vi "Tic Tac Toe - Without Event.vi"() -> ()   [LabVIEW 2022 SP3]
panel:
  in  "B 9":bool
  in  "B 8":bool
  in  "B 7":bool
  in  "B 6":bool
  in  "B 5":bool
  in  "B 4":bool
  in  "B 3":bool
  in  "B 2":bool
  in  "B 1":bool
  in  "Exit":bool
  in  "Reset":bool
  in  "Start Game":bool
  out "Player 2 Symbol":u16(ring)
  in  "Player 2 Name":string="Steve"
  out "Player 1 Symbol":u16(ring)
  in  "Player 1 Name":string="Mark"
  in  "9":u16(ring)
  in  "8":u16(ring)
  in  "7":u16(ring)
  in  "6":u16(ring)
  in  "5":u16(ring)
  in  "4":u16(ring)
  in  "3":u16(ring)
  in  "2":u16(ring)
  in  "1":u16(ring)
  # "TIC TAC TOE"
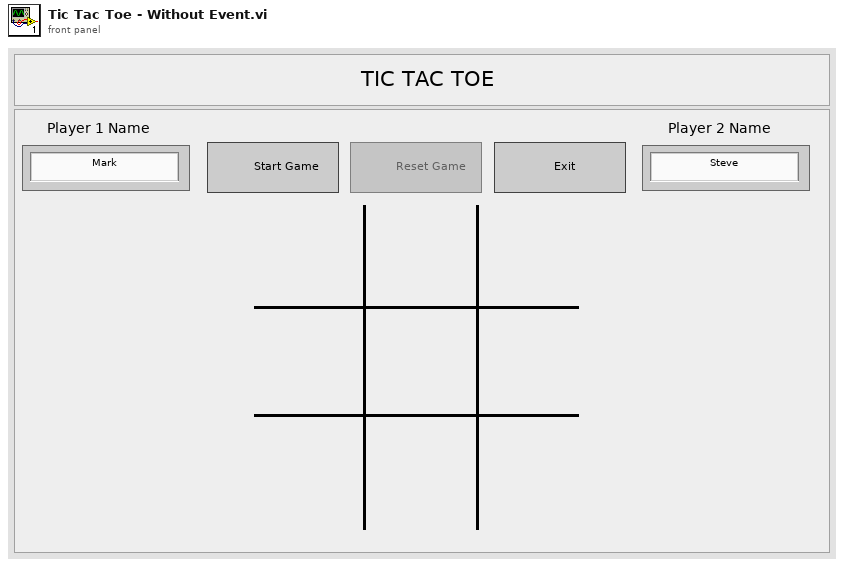
[diagram p1: front panel]
types:
  T1 = enum8{"Enabled", "Disabled", "Disabled and Grayed Out"}
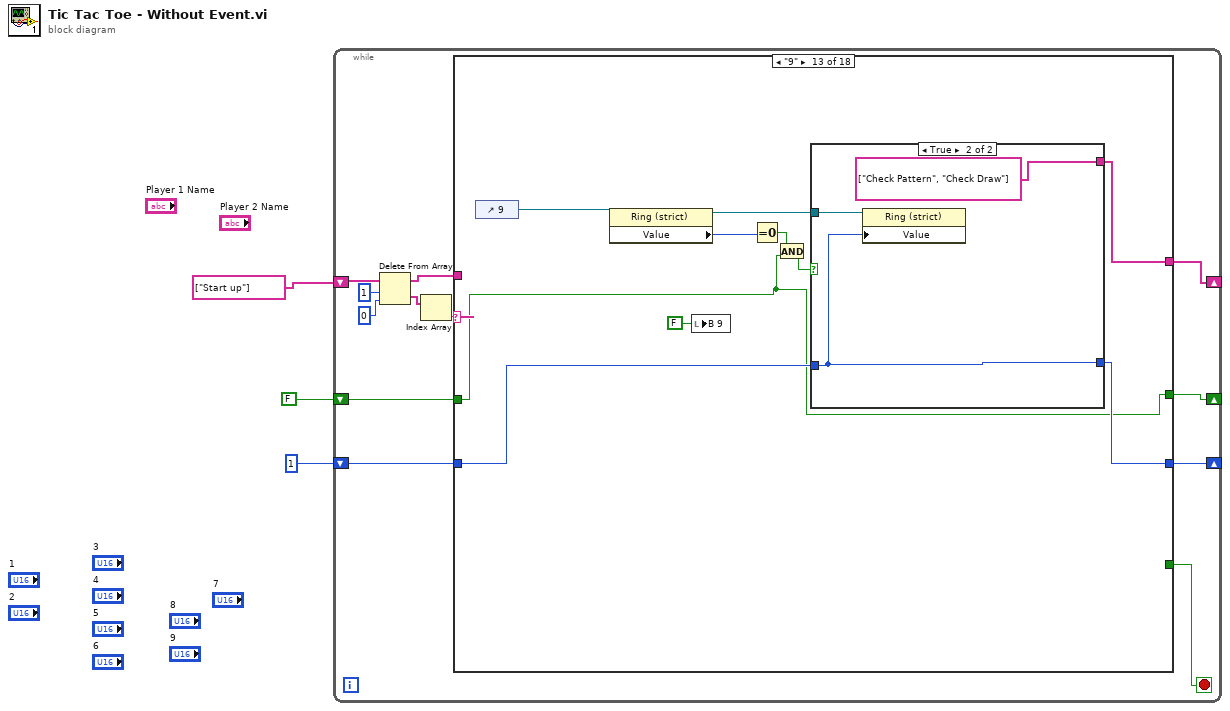
[diagram p0: block diagram]
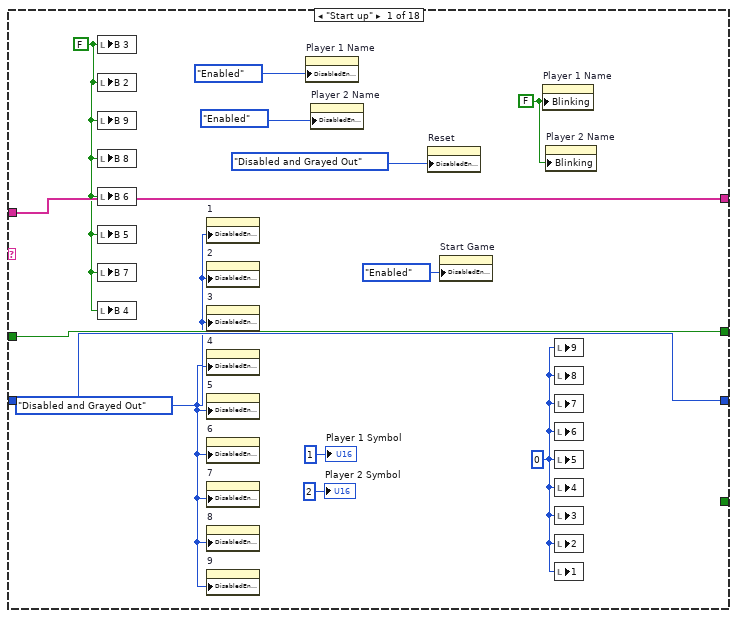
[diagram p2: hidden frame]
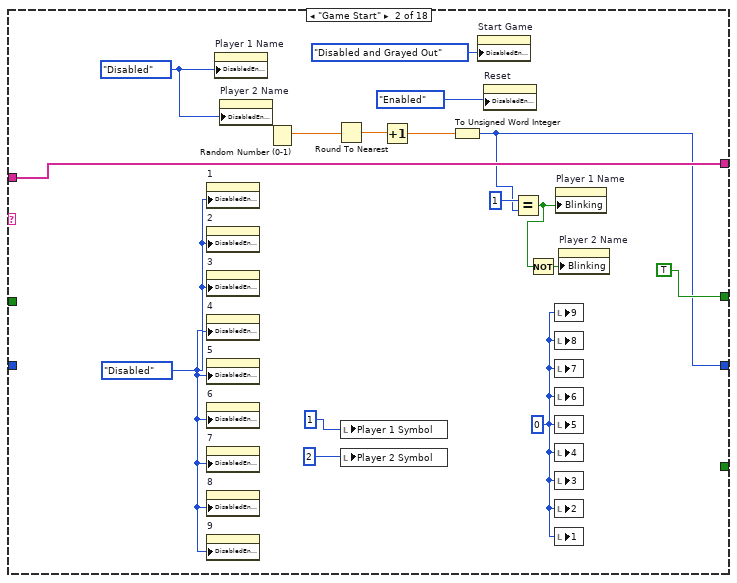
[diagram p3: hidden frame]
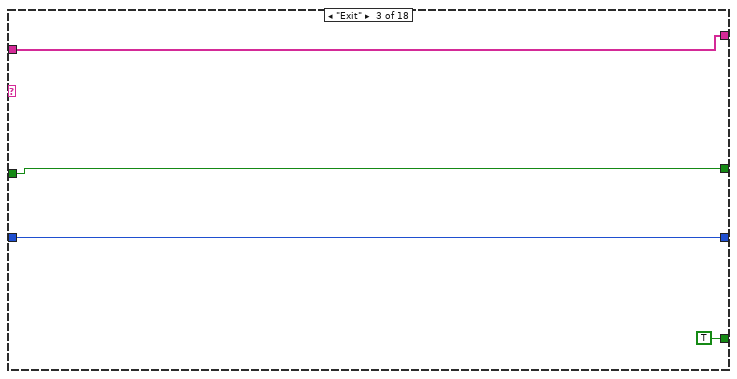
[diagram p4: hidden frame]
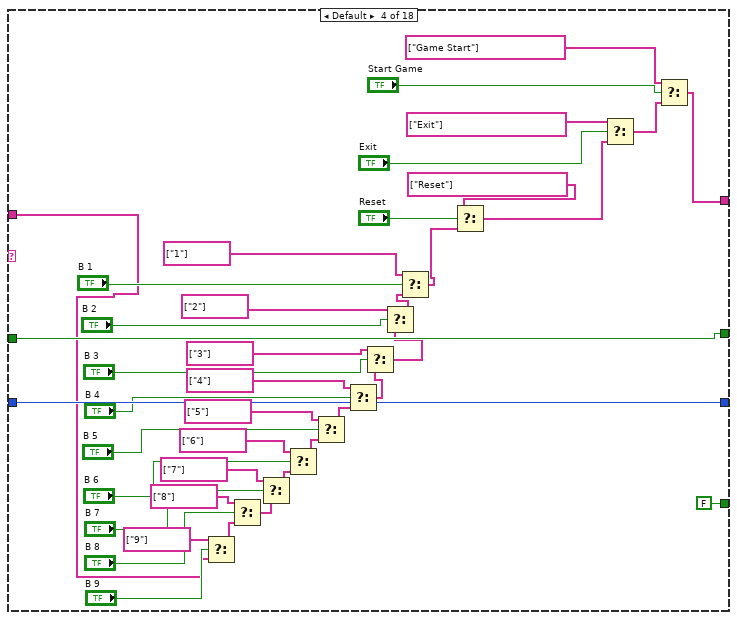
[diagram p5: hidden frame]
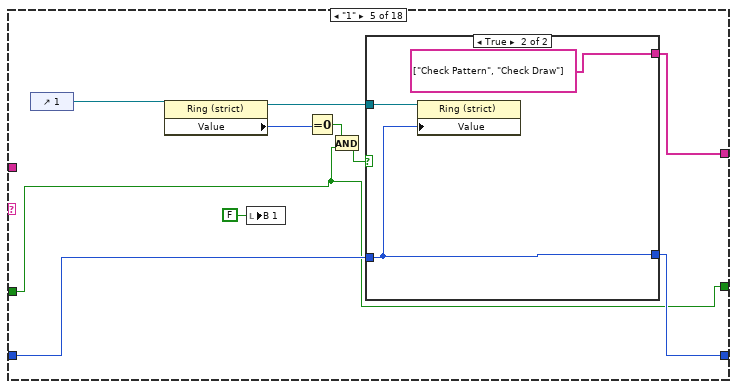
[diagram p6: hidden frame]
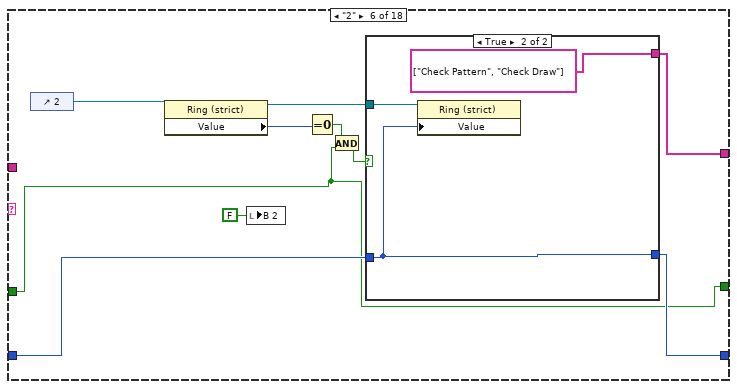
[diagram p8: hidden frame]
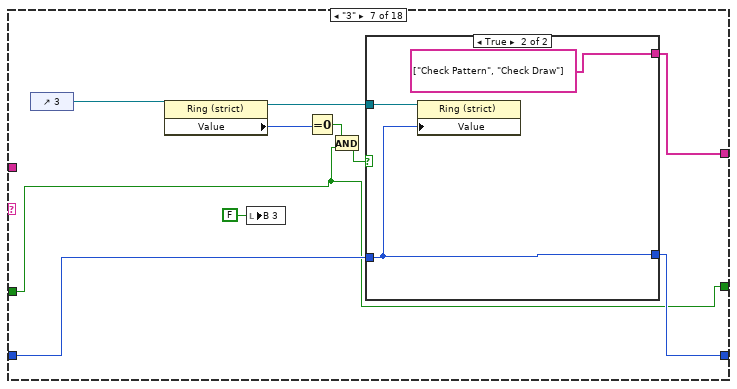
[diagram p10: hidden frame]
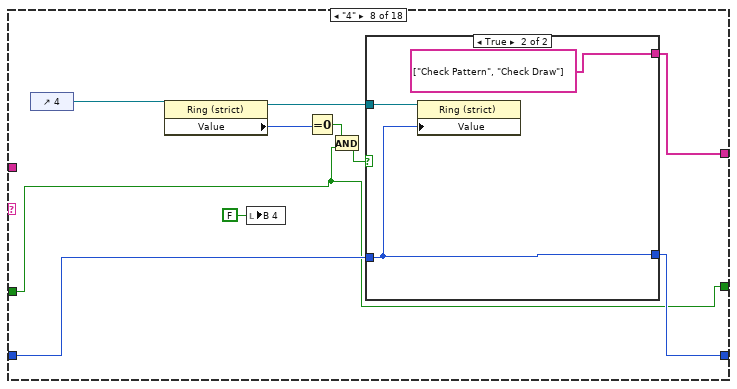
[diagram p12: hidden frame]
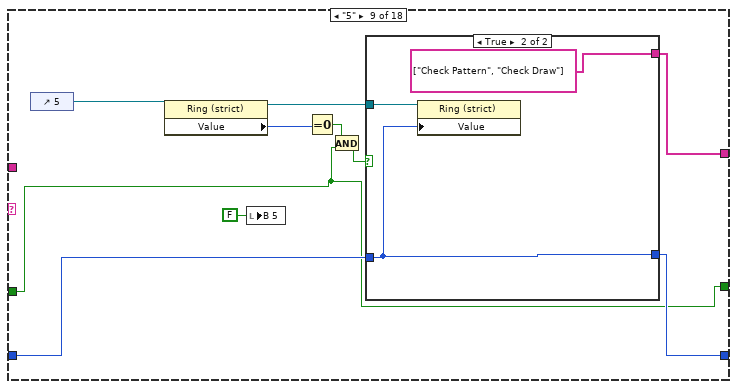
[diagram p14: hidden frame]
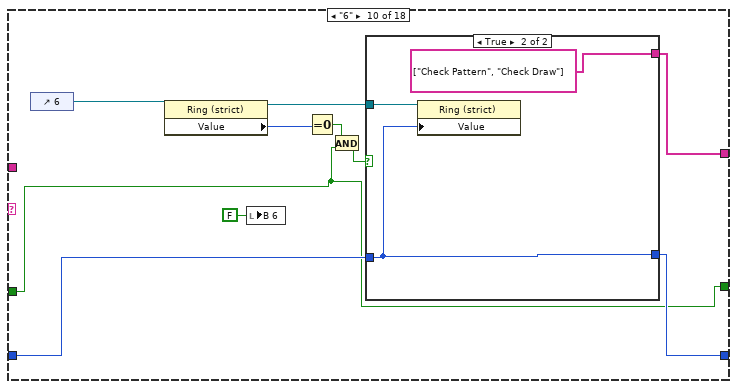
[diagram p16: hidden frame]
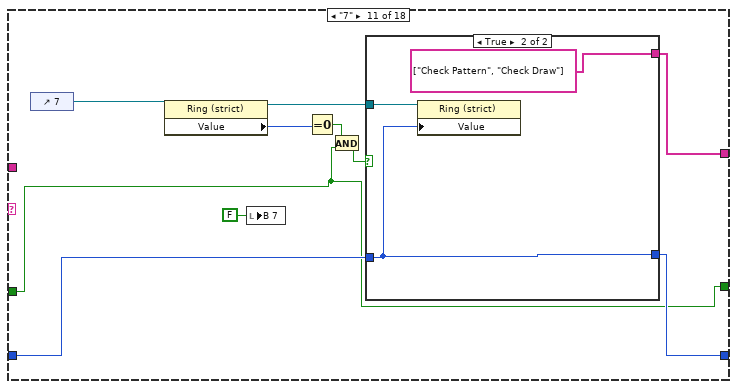
[diagram p18: hidden frame]
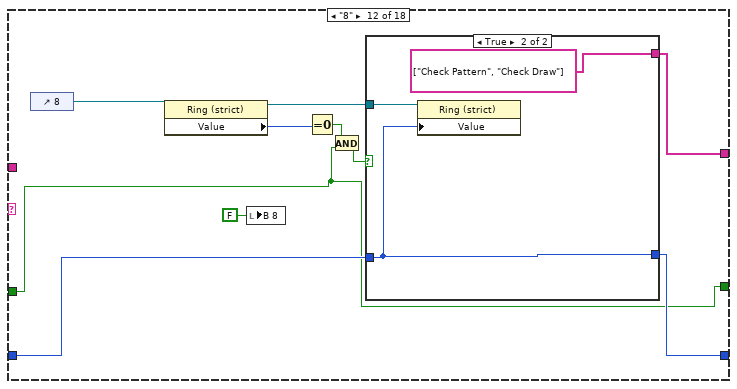
[diagram p20: hidden frame]
diagram:
  n1 = while {
    shift-right: [w10] -> _
    shift-left: string[] ["Start up"] -> [w15]
    shift-right: [w8] -> _
    shift-left: FALSE -> [w7]
    shift-right: [w6] -> _
    shift-left: u16 1 ("9") -> [w5]
    stop <- w4 stop-if-true
    n2 = Delete From Array(array=w15, length=1, index=0) -> (deleted portion=w12:string[], array with subset deleted=w9:string[])
    n3 = Index Array(array=w12) -> (element=w11:string)  [unwired: 1 in]
    n4 = case shown="\"9\"" w11 {
      tunnel: [w28 w44 w45 w83 w94 w108 w122 w136 w150 w164 w178 w192 w206 w217 w224 w276 string[] ["Start up"] string[] ["Start up"]] -> w10
      tunnel: w9 -> [w28 w44 w45 w65 _ _ _ _ _ _ _ _ _ w218 w225 w277 _ _]
      tunnel: [w24 TRUE w46 w87 w90 w104 w118 w132 w146 w160 w174 w188 w202 w216 w261 w291 FALSE FALSE] -> w8
      tunnel: w7 -> [w24 _ w46 w87 w90 w104 w118 w132 w146 w160 w174 w188 w202 w216 w261 w291 _ _]
      tunnel: [w23 w29 w47 w88 w91 w105 w119 w133 w147 w161 w175 w189 w203 w215 w223 w269 w300 w302] -> w6
      tunnel: w5 -> [w23 _ w47 w88 w92 w106 w120 w134 w148 w162 w176 w190 w204 w215 w223 w275 w300 w302]
      tunnel: [_ _ TRUE FALSE _ _ _ _ _ _ _ _ _ _ _ _ _ _] -> w4
      frame "Start up" {
        w16 = FALSE ("B 3")
        w20 = FALSE ("Blinking")
        w22 = T1."Disabled and Grayed Out" ("Disabled")
        w27 = u16 0 ("9")
        n5 = local write "B 3"(w16) -> ()
        n6 = local write "B 2"(w16) -> ()
        n7 = local write "B 9"(w16) -> ()
        n8 = local write "B 8"(w16) -> ()
        n9 = local write "B 6"(w16) -> ()
        n10 = local write "B 5"(w16) -> ()
        n11 = local write "B 7"(w16) -> ()
        n12 = local write "B 4"(w16) -> ()
        n13 = property on="1" class="Ring (strict)"("DisabledEnum"=w22) -> ()  [unwired: 2 in, 2 out]
        n14 = property on="2" class="Ring (strict)"("DisabledEnum"=w22) -> ()  [unwired: 2 in, 2 out]
        n15 = property on="3" class="Ring (strict)"("DisabledEnum"=w22) -> ()  [unwired: 2 in, 2 out]
        n16 = property on="4" class="Ring (strict)"("DisabledEnum"=w22) -> ()  [unwired: 2 in, 2 out]
        n17 = property on="5" class="Ring (strict)"("DisabledEnum"=w22) -> ()  [unwired: 2 in, 2 out]
        n18 = property on="6" class="Ring (strict)"("DisabledEnum"=w22) -> ()  [unwired: 2 in, 2 out]
        n19 = property on="7" class="Ring (strict)"("DisabledEnum"=w22) -> ()  [unwired: 2 in, 2 out]
        n20 = property on="8" class="Ring (strict)"("DisabledEnum"=w22) -> ()  [unwired: 2 in, 2 out]
        n21 = property on="9" class="Ring (strict)"("DisabledEnum"=w22) -> ()  [unwired: 2 in, 2 out]
        n22 = property on="Player 1 Name" class="Str"("DisabledEnum"=T1."Enabled" ("Disabled")) -> ()  [unwired: 2 in, 2 out]
        n23 = property on="Player 2 Name" class="Str"("DisabledEnum"=T1."Enabled" ("Disabled")) -> ()  [unwired: 2 in, 2 out]
        n24 = property on="Reset" class="Bool"("DisabledEnum"=T1."Disabled and Grayed Out" ("Disabled")) -> ()  [unwired: 2 in, 2 out]
        n25 = property on="Start Game" class="Bool"("DisabledEnum"=T1."Enabled" ("Disabled")) -> ()  [unwired: 2 in, 2 out]
        n26 = property on="Player 1 Name" class="Str"("Blinking"=w20) -> ()  [unwired: 2 in, 2 out]
        n27 = property on="Player 2 Name" class="Str"("Blinking"=w20) -> ()  [unwired: 2 in, 2 out]
        n28 = local write "9"(w27) -> ()
        n29 = local write "8"(w27) -> ()
        n30 = local write "7"(w27) -> ()
        n31 = local write "6"(w27) -> ()
        n32 = local write "5"(w27) -> ()
        n33 = local write "4"(w27) -> ()
        n34 = local write "3"(w27) -> ()
        n35 = local write "2"(w27) -> ()
        n36 = local write "1"(w27) -> ()
        "Player 1 Symbol" <- u16 1 ("Player 1 Symbol")
        "Player 2 Symbol" <- u16 2 ("Player 2 Symbol")
      }
      frame "Game Start" {
        w37 = T1."Disabled" ("Disabled")
        w42 = T1."Disabled" ("Disabled")
        w43 = u16 0 ("9")
        n37 = property on="1" class="Ring (strict)"("DisabledEnum"=w42) -> ()  [unwired: 2 in, 2 out]
        n38 = property on="2" class="Ring (strict)"("DisabledEnum"=w42) -> ()  [unwired: 2 in, 2 out]
        n39 = property on="3" class="Ring (strict)"("DisabledEnum"=w42) -> ()  [unwired: 2 in, 2 out]
        n40 = property on="4" class="Ring (strict)"("DisabledEnum"=w42) -> ()  [unwired: 2 in, 2 out]
        n41 = property on="5" class="Ring (strict)"("DisabledEnum"=w42) -> ()  [unwired: 2 in, 2 out]
        n42 = property on="6" class="Ring (strict)"("DisabledEnum"=w42) -> ()  [unwired: 2 in, 2 out]
        n43 = property on="7" class="Ring (strict)"("DisabledEnum"=w42) -> ()  [unwired: 2 in, 2 out]
        n44 = property on="8" class="Ring (strict)"("DisabledEnum"=w42) -> ()  [unwired: 2 in, 2 out]
        n45 = property on="9" class="Ring (strict)"("DisabledEnum"=w42) -> ()  [unwired: 2 in, 2 out]
        n46 = property on="Player 1 Name" class="Str"("DisabledEnum"=w37) -> ()  [unwired: 2 in, 2 out]
        n47 = property on="Player 2 Name" class="Str"("DisabledEnum"=w37) -> ()  [unwired: 2 in, 2 out]
        n48 = Random Number (0-1)() -> (number: 0 to 1=w30:dbl)
        n49 = Round To Nearest(number=w30) -> (nearest integer value=w31:dbl)
        n50 = local write "Player 1 Symbol"(u16 1 ("Player 1 Symbol")) -> ()
        n51 = local write "Player 2 Symbol"(u16 2 ("Player 2 Symbol")) -> ()
        n52 = Increment(x=w31) -> (x+1=w32:dbl)
        n53 = To Unsigned Word Integer(number=w32) -> (unsigned 16bit integer=w29:u16)
        n54 = property on="Start Game" class="Bool"("DisabledEnum"=T1."Disabled and Grayed Out" ("Disabled")) -> ()  [unwired: 2 in, 2 out]
        n55 = property on="Reset" class="Bool"("DisabledEnum"=T1."Enabled" ("Disabled")) -> ()  [unwired: 2 in, 2 out]
        n56 = Equal?(x=u16 1, y=w29) -> (x = y?=w35:bool)
        n57 = Not(x=w35) -> (.not. x?=w34:bool)
        n58 = local write "9"(w43) -> ()
        n59 = local write "8"(w43) -> ()
        n60 = local write "7"(w43) -> ()
        n61 = local write "6"(w43) -> ()
        n62 = local write "5"(w43) -> ()
        n63 = local write "4"(w43) -> ()
        n64 = local write "3"(w43) -> ()
        n65 = local write "2"(w43) -> ()
        n66 = local write "1"(w43) -> ()
        n67 = property on="Player 1 Name" class="Str"("Blinking"=w35) -> ()  [unwired: 2 in, 2 out]
        n68 = property on="Player 2 Name" class="Str"("Blinking"=w34) -> ()  [unwired: 2 in, 2 out]
      }
      frame "Exit" {
      }
      frame Default {
        n69 = Select(t=string[] ["9"], s="B 9", f=w65) -> (s? t:f=w57:string[])
        n70 = Select(t=string[] ["8"], s="B 8", f=w57) -> (s? t:f=w58:string[])
        n71 = Select(t=string[] ["7"], s="B 7", f=w58) -> (s? t:f=w59:string[])
        n72 = Select(t=string[] ["6"], s="B 6", f=w59) -> (s? t:f=w60:string[])
        n73 = Select(t=string[] ["5"], s="B 5", f=w60) -> (s? t:f=w61:string[])
        n74 = Select(t=string[] ["4"], s="B 4", f=w61) -> (s? t:f=w62:string[])
        n75 = Select(t=string[] ["3"], s="B 3", f=w62) -> (s? t:f=w63:string[])
        n76 = Select(t=string[] ["2"], s="B 2", f=w63) -> (s? t:f=w64:string[])
        n77 = Select(t=string[] ["1"], s="B 1", f=w64) -> (s? t:f=w74:string[])
        n78 = Select(t=string[] ["Reset"], s="Reset", f=w74) -> (s? t:f=w77:string[])
        n79 = Select(t=string[] ["Exit"], s="Exit", f=w77) -> (s? t:f=w80:string[])
        n80 = Select(t=string[] ["Game Start"], s="Start Game", f=w80) -> (s? t:f=w83:string[])
      }
      frame "1" {
        n81 = control-ref of="1"() -> (w93:refnum<vi>)
        n82 = property class="Ring (strict)"(reference=w93) -> (reference out=w96:refnum<vi>, "Value"=w95:u16)  [unwired: 1 in, 1 out]
        n83 = local write "B 1"(FALSE ("B 1")) -> ()
        n84 = Equal To 0?(x=w95) -> (x = 0?=w97:bool)
        n85 = And(x=w97, y=w90) -> (x .and. y?=w98:bool)
        n86 = case shown="True" w98 {
          tunnel: [_ string[] ["Check Pattern", "Check Draw"]] -> w94
          tunnel: w92 -> [w99 w100]
          tunnel: [w99 w100] -> w91
          tunnel: w96 -> [_ w101]
          frame False {
          }
          frame True {
            n87 = property class="Ring (strict)"(reference=w101, "Value"=w100) -> ()  [unwired: 1 in, 2 out]
          }
        }
      }
      frame "2" {
        n88 = control-ref of="2"() -> (w107:refnum<vi>)
        n89 = property class="Ring (strict)"(reference=w107) -> (reference out=w110:refnum<vi>, "Value"=w109:u16)  [unwired: 1 in, 1 out]
        n90 = local write "B 2"(FALSE ("B 1")) -> ()
        n91 = Equal To 0?(x=w109) -> (x = 0?=w111:bool)
        n92 = And(x=w111, y=w104) -> (x .and. y?=w112:bool)
        n93 = case shown="True" w112 {
          tunnel: [_ string[] ["Check Pattern", "Check Draw"]] -> w108
          tunnel: w106 -> [w113 w114]
          tunnel: [w113 w114] -> w105
          tunnel: w110 -> [_ w115]
          frame False {
          }
          frame True {
            n94 = property class="Ring (strict)"(reference=w115, "Value"=w114) -> ()  [unwired: 1 in, 2 out]
          }
        }
      }
      frame "3" {
        n95 = control-ref of="3"() -> (w121:refnum<vi>)
        n96 = property class="Ring (strict)"(reference=w121) -> (reference out=w124:refnum<vi>, "Value"=w123:u16)  [unwired: 1 in, 1 out]
        n97 = local write "B 3"(FALSE ("B 1")) -> ()
        n98 = Equal To 0?(x=w123) -> (x = 0?=w125:bool)
        n99 = And(x=w125, y=w118) -> (x .and. y?=w126:bool)
        n100 = case shown="True" w126 {
          tunnel: [_ string[] ["Check Pattern", "Check Draw"]] -> w122
          tunnel: w120 -> [w127 w128]
          tunnel: [w127 w128] -> w119
          tunnel: w124 -> [_ w129]
          frame False {
          }
          frame True {
            n101 = property class="Ring (strict)"(reference=w129, "Value"=w128) -> ()  [unwired: 1 in, 2 out]
          }
        }
      }
      frame "4" {
        n102 = control-ref of="4"() -> (w135:refnum<vi>)
        n103 = property class="Ring (strict)"(reference=w135) -> (reference out=w138:refnum<vi>, "Value"=w137:u16)  [unwired: 1 in, 1 out]
        n104 = local write "B 4"(FALSE ("B 1")) -> ()
        n105 = Equal To 0?(x=w137) -> (x = 0?=w139:bool)
        n106 = And(x=w139, y=w132) -> (x .and. y?=w140:bool)
        n107 = case shown="True" w140 {
          tunnel: [_ string[] ["Check Pattern", "Check Draw"]] -> w136
          tunnel: w134 -> [w141 w142]
          tunnel: [w141 w142] -> w133
          tunnel: w138 -> [_ w143]
          frame False {
          }
          frame True {
            n108 = property class="Ring (strict)"(reference=w143, "Value"=w142) -> ()  [unwired: 1 in, 2 out]
          }
        }
      }
      frame "5" {
        n109 = control-ref of="5"() -> (w149:refnum<vi>)
        n110 = property class="Ring (strict)"(reference=w149) -> (reference out=w152:refnum<vi>, "Value"=w151:u16)  [unwired: 1 in, 1 out]
        n111 = local write "B 5"(FALSE ("B 1")) -> ()
        n112 = Equal To 0?(x=w151) -> (x = 0?=w153:bool)
        n113 = And(x=w153, y=w146) -> (x .and. y?=w154:bool)
        n114 = case shown="True" w154 {
          tunnel: [_ string[] ["Check Pattern", "Check Draw"]] -> w150
          tunnel: w148 -> [w155 w156]
          tunnel: [w155 w156] -> w147
          tunnel: w152 -> [_ w157]
          frame False {
          }
          frame True {
            n115 = property class="Ring (strict)"(reference=w157, "Value"=w156) -> ()  [unwired: 1 in, 2 out]
          }
        }
      }
      frame "6" {
        n116 = control-ref of="6"() -> (w163:refnum<vi>)
        n117 = property class="Ring (strict)"(reference=w163) -> (reference out=w166:refnum<vi>, "Value"=w165:u16)  [unwired: 1 in, 1 out]
        n118 = local write "B 6"(FALSE ("B 1")) -> ()
        n119 = Equal To 0?(x=w165) -> (x = 0?=w167:bool)
        n120 = And(x=w167, y=w160) -> (x .and. y?=w168:bool)
        n121 = case shown="True" w168 {
          tunnel: [_ string[] ["Check Pattern", "Check Draw"]] -> w164
          tunnel: w162 -> [w169 w170]
          tunnel: [w169 w170] -> w161
          tunnel: w166 -> [_ w171]
          frame False {
          }
          frame True {
            n122 = property class="Ring (strict)"(reference=w171, "Value"=w170) -> ()  [unwired: 1 in, 2 out]
          }
        }
      }
      frame "7" {
        n123 = control-ref of="7"() -> (w177:refnum<vi>)
        n124 = property class="Ring (strict)"(reference=w177) -> (reference out=w180:refnum<vi>, "Value"=w179:u16)  [unwired: 1 in, 1 out]
        n125 = local write "B 7"(FALSE ("B 1")) -> ()
        n126 = Equal To 0?(x=w179) -> (x = 0?=w181:bool)
        n127 = And(x=w181, y=w174) -> (x .and. y?=w182:bool)
        n128 = case shown="True" w182 {
          tunnel: [_ string[] ["Check Pattern", "Check Draw"]] -> w178
          tunnel: w176 -> [w183 w184]
          tunnel: [w183 w184] -> w175
          tunnel: w180 -> [_ w185]
          frame False {
          }
          frame True {
            n129 = property class="Ring (strict)"(reference=w185, "Value"=w184) -> ()  [unwired: 1 in, 2 out]
          }
        }
      }
      frame "8" {
        n130 = control-ref of="8"() -> (w191:refnum<vi>)
        n131 = property class="Ring (strict)"(reference=w191) -> (reference out=w194:refnum<vi>, "Value"=w193:u16)  [unwired: 1 in, 1 out]
        n132 = local write "B 8"(FALSE ("B 1")) -> ()
        n133 = Equal To 0?(x=w193) -> (x = 0?=w195:bool)
        n134 = And(x=w195, y=w188) -> (x .and. y?=w196:bool)
        n135 = case shown="True" w196 {
          tunnel: [_ string[] ["Check Pattern", "Check Draw"]] -> w192
          tunnel: w190 -> [w197 w198]
          tunnel: [w197 w198] -> w189
          tunnel: w194 -> [_ w199]
          frame False {
          }
          frame True {
            n136 = property class="Ring (strict)"(reference=w199, "Value"=w198) -> ()  [unwired: 1 in, 2 out]
          }
        }
      }
      frame "9" {
        n137 = control-ref of="9"() -> (w205:refnum<vi>)
        n138 = property class="Ring (strict)"(reference=w205) -> (reference out=w208:refnum<vi>, "Value"=w207:u16)  [unwired: 1 in, 1 out]
        n139 = local write "B 9"(FALSE ("B 1")) -> ()
        n140 = Equal To 0?(x=w207) -> (x = 0?=w209:bool)
        n141 = And(x=w209, y=w202) -> (x .and. y?=w210:bool)
        n142 = case shown="True" w210 {
          tunnel: [_ string[] ["Check Pattern", "Check Draw"]] -> w206
          tunnel: w204 -> [w211 w212]
          tunnel: [w211 w212] -> w203
          tunnel: w208 -> [_ w213]
          frame False {
          }
          frame True {
            n143 = property class="Ring (strict)"(reference=w213, "Value"=w212) -> ()  [unwired: 1 in, 2 out]
          }
        }
      }
      frame "Reset" {
        n144 = Two Button Dialog(message="Do you want to Reset the Game?") -> (T button?=w220:bool)  [unwired: 2 in]
        n145 = Select(t=string[] ["Start up"], s=w220, f=w218) -> (s? t:f=w217:string[])
      }
      frame "Check Pattern" {
        n146 = local read "1"() -> (w256:u16)
        n147 = local read "2"() -> (w255:u16)
        n148 = local read "3"() -> (w254:u16)
        n149 = local read "1"() -> (w242:u16)
        n150 = local read "4"() -> (w241:u16)
        n151 = local read "7"() -> (w240:u16)
        n152 = local read "1"() -> (w239:u16)
        n153 = local read "5"() -> (w238:u16)
        n154 = local read "9"() -> (w237:u16)
        n155 = local read "4"() -> (w253:u16)
        n156 = local read "5"() -> (w252:u16)
        n157 = local read "6"() -> (w251:u16)
        n158 = local read "2"() -> (w245:u16)
        n159 = local read "5"() -> (w244:u16)
        n160 = local read "8"() -> (w243:u16)
        n161 = local read "3"() -> (w236:u16)
        n162 = local read "5"() -> (w235:u16)
        n163 = local read "7"() -> (w234:u16)
        n164 = local read "7"() -> (w250:u16)
        n165 = local read "8"() -> (w249:u16)
        n166 = local read "9"() -> (w248:u16)
        n167 = local read "3"() -> (w247:u16)
        n168 = local read "6"() -> (w246:u16)
        n169 = local read "9"() -> (w222:u16)
        n170 = Build Array(w256, w255, w254) -> (w233:u16[])
        n171 = Build Array(w242, w241, w240) -> (w232:u16[])
        n172 = Build Array(w239, w238, w237) -> (w231:u16[])
        n173 = Build Array(w253, w252, w251) -> (w230:u16[])
        n174 = Build Array(w245, w244, w243) -> (w229:u16[])
        n175 = Build Array(w236, w235, w234) -> (w228:u16[])
        n176 = Build Array(w250, w249, w248) -> (w227:u16[])
        n177 = Build Array(w247, w246, w222) -> (w226:u16[])
        n178 = Build Array(w233, w232, w231, w230, w229, w228, w227, w226) -> (w257:u16[][])
        n179 = for {
          tunnel: w257 -> [w265] mode=indexing
          tunnel: w223 -> [w264]
          tunnel: [w262] -> w258
          stop <- w262 stop-if-true
          n180 = for {
            tunnel: w265 -> [w268] mode=indexing
            tunnel: w264 -> [w267]
            tunnel: [w266] -> w263 mode=indexing
            n181 = Equal?(x=w268, y=w267) -> (x = y?=w266:bool)
          }
          n182 = And Array Elements(Boolean array=w263) -> (logical AND=w262:bool)
        }
        n183 = Build Array("Match Won") -> (w260:string[])
        n184 = Select(t=w260, s=w258, f=w225) -> (s? t:f=w224:string[])
      }
      frame "Check Draw" {
        n185 = local read "1"() -> (w290:u16)
        n186 = local read "2"() -> (w289:u16)
        n187 = local read "3"() -> (w288:u16)
        n188 = local read "4"() -> (w287:u16)
        n189 = local read "5"() -> (w286:u16)
        n190 = local read "6"() -> (w285:u16)
        n191 = local read "7"() -> (w284:u16)
        n192 = local read "8"() -> (w283:u16)
        n193 = local read "9"() -> (w282:u16)
        n194 = Build Array(w290, w289, w288, w287, w286, w285, w284, w283, w282) -> (w281:u16[])
        n195 = for {
          tunnel: w281 -> [w297] mode=indexing
          tunnel: [w296] -> w280 mode=indexing
          n196 = Not Equal To 0?(x=w297) -> (x != 0?=w296:bool)
        }
        n197 = Equal?(x=u16 1, y=w275) -> (x = y?=w271:bool)
        n198 = Select(t=u16 2 ("9"), s=w271, f=u16 1 ("9")) -> (s? t:f=w269:u16)
        n199 = And Array Elements(Boolean array=w280) -> (logical AND=w270:bool)
        n200 = case shown="False" w270 {
          tunnel: w269 -> [w294 _]
          frame False {
            n201 = Equal?(x=u16 1, y=w294) -> (x = y?=w292:bool)
            n202 = Not(x=w292) -> (.not. x?=w293:bool)
            n203 = property on="Player 1 Name" class="Str"("Blinking"=w292) -> ()  [unwired: 2 in, 2 out]
            n204 = property on="Player 2 Name" class="Str"("Blinking"=w293) -> ()  [unwired: 2 in, 2 out]
          }
          frame True {
          }
        }
        n205 = Build Array("Match Draw") -> (w279:string[])
        n206 = Select(t=w279, s=w270, f=w277) -> (s? t:f=w276:string[])
      }
      frame "Match Draw" {
        n207 = One Button Dialog(message="Match Drawn") -> ()  [unwired: 1 in, 1 out]
      }
      frame "Match Won" {
        n208 = Format Into String(format string="Player %d Win !!" ("message"), w302) -> (resulting string=w304:string)  [unwired: 2 in, 1 out]
        n209 = One Button Dialog(message=w304) -> ()  [unwired: 1 in, 1 out]
      }
    }
  }
